vi "Data Get Byte Array.vi"(8 "error in (no error)":errorcluster, 11 "Data DVR in":refnum<data-value>) -> (0 "error out":errorcluster, 1 "Array dimensions":i32[](array[numeric]), 2 "I8 array out":i8[](array[numeric]), 3 "Data DVR out":refnum<data-value>)   [LabVIEW 2010, in "MDSplus.lvlib"]
doc: "Converts this data into a byte array. Implemented at this class level by returning TDI data(BYTE(this)). If data() fails or the returned class is not array, it generates an exception. It will return a 1 dimensional array using row-first ordering if a multidimensional array."
uses:
  <vilib>/MDSplus/Library/MDSplus.lvlib
  <vilib>/MDSplus/Classes/Data_Class/Data.lvclass
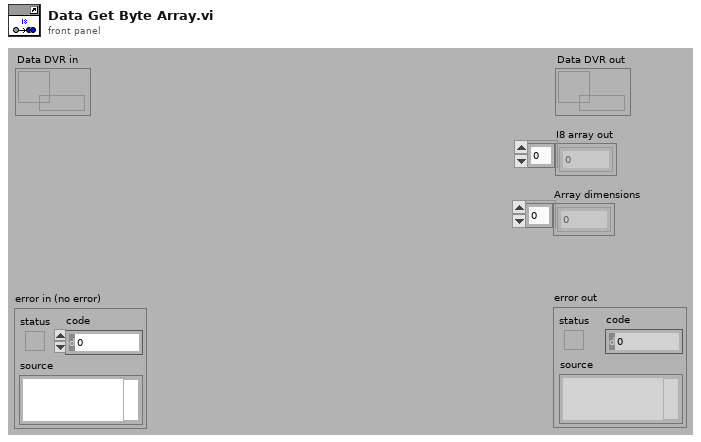
[diagram p1: front panel]
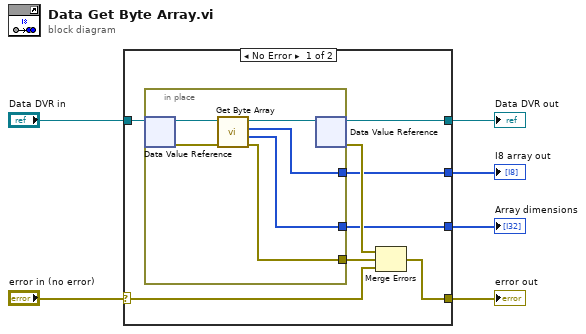
[diagram p0: block diagram]
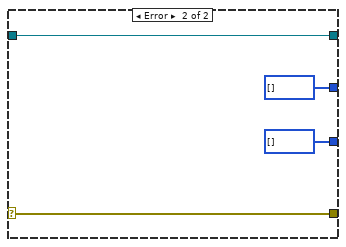
[diagram p2: hidden frame]
diagram:
  n1 = case shown="No Error" "error in (no error)" {
    selector: "error in (no error)" -> [w12 w24]
    tunnel: "Data DVR in" -> [w14 w23]
    tunnel: [w10 w24] -> w6
    tunnel: [w9 w23] -> w3
    tunnel: [w8 i8[] [] ("SGL array out")] -> w2
    tunnel: [w7 i32[] [] ("Array dimensions")] -> w1
    frame No Error {
      n2 = in-place {
        in-place-border: [w18] -> w13
        in-place-border: [w16] -> w8
        in-place-border: [w15] -> w7
        n3 = in-place-dvr #1(w14) -> (w20:refnum<class "Data.lvclass">, w17:errorcluster)
        n4 = call-dynamic "Get Byte Array.vi"("error in (no error)"=w17, "Data in"=w20) -> ("error out"=w18:errorcluster, "Array dimensions"=w15:i32[], "I8 array out"=w16:i8[], "Data out"=w19:refnum<class "Data.lvclass">)  [unwired: 6 in]
        n5 = in-place-dvr #1(w19) -> (w9:refnum<data-value>, w11:errorcluster)
      }
      n6 = Merge Errors(w11, w13, w12) -> (w10:errorcluster)
    }
    frame Error {
    }
  }
  "error out" <- w6
  "Data DVR out" <- w3
  "I8 array out" <- w2
  "Array dimensions" <- w1
